vi "OAT Validate Spectrogram Config.vi"(11 "config":T1={"type"=enum."Order-RPM", "range"={"start"=0.0, "end"=0.0, "step"=0.0}} {"range"."step" format="%.2f"; "range"."end" format="%.2f"; "range"."start" format="%.2f"}) -> (3 "config":T1={"type"=enum."Order-RPM", "range"={"start"=0.0, "end"=0.0, "step"=0.0}} {"range"."step" format="%.2f"; "range"."end" format="%.2f"; "range"."start" format="%.2f"})   [LabVIEW 2017, in "SoundVib_Resampling.lvlib"]
uses:
  <vilib>/addons/Sound and Vibration/Order Analysis/Resample Order Tracking/SoundVib_Resampling.lvlib
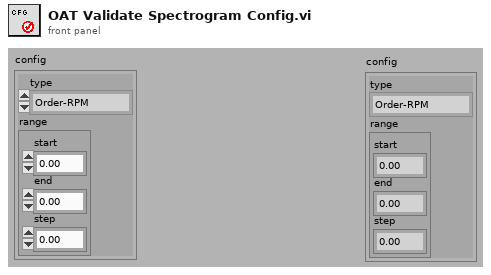
[diagram p1: front panel]
types:
  T1 = cluster{"type":enum16{"Frequency-Time", "Frequency-RPM", "Order-RPM"}, "range":cluster{"start":dbl, "end":dbl, "step":dbl}}
  T2 = enum16{"Frequency-Time", "Frequency-RPM", "Order-RPM"}
  T3 = enum16{"Frequency-Time", "Frequency-RPM", "Order-RPM", "RPM-Order"}
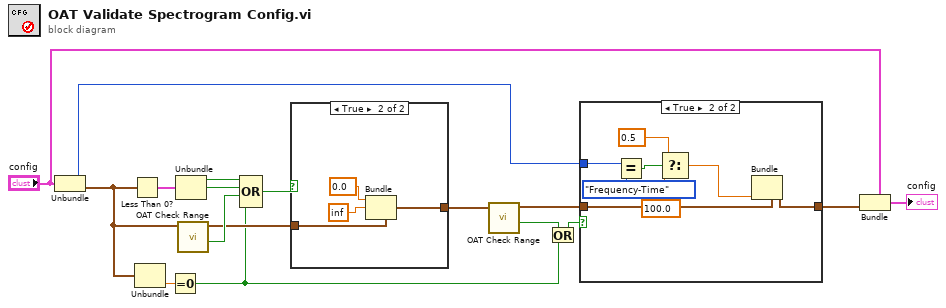
[diagram p0: block diagram]
diagram:
  n1 = Unbundle("config") -> ("type"=w10:T2, "range"=w2:cluster{"start":dbl, "end":dbl, "step":dbl})
  n2 = Less Than 0?(x=w2) -> (x < 0?=w17:cluster{"start":bool, "end":bool, "step":bool})
  n3 = Unbundle(w2) -> ("step"=w6:dbl)  [unwired: 2 out]
  n4 = Equal To 0?(x=w6) -> (x = 0?=w1:bool)
  n5 = Unbundle(w17) -> ("start"=w16:bool, "end"=w15:bool)  [unwired: 1 out]
  n6 = call <vilib>:"OAT Check Range.vi"("range in"=w2) -> ("empty?"=w14:bool, "range out"=w12:cluster{"start":dbl, "end":dbl, "step":dbl})  [unwired: 8 in, 1 out]
  n7 = Compound Arithmetic op=OR(w16, w15, w14, w1) -> (w13:bool)
  n8 = case shown="True" w13 {
    tunnel: w12 -> [w18 w22]
    tunnel: [w18 w19] -> w3
    frame False {
    }
    frame True {
      n9 = Bundle(cluster=w22, "start"=0.0, "end"=inf) -> (w19:cluster{"start":dbl, "end":dbl, "step":dbl})  [unwired: 1 in]
    }
  }
  n10 = call <vilib>:"OAT Check Range.vi"("range in"=w3) -> ("empty?"=w5:bool, "range out"=w11:cluster{"start":dbl, "end":dbl, "step":dbl})  [unwired: 8 in, 1 out]
  n11 = Or(x=w5, y=w1) -> (x .or. y?=w4:bool)
  n12 = case shown="True" w4 {
    tunnel: w11 -> [w23 w26]
    tunnel: [w23 w25] -> w9
    tunnel: w10 -> [_ w30]
    frame False {
    }
    frame True {
      n13 = Equal?(x=w30, y=T3."Frequency-Time") -> (x = y?=w31:bool)
      n14 = Select(t=0.5, s=w31, f=100.0) -> (s? t:f=w24:dbl)
      n15 = Bundle(cluster=w26, "step"=w24) -> (w25:cluster{"start":dbl, "end":dbl, "step":dbl})  [unwired: 2 in]
    }
  }
  n16 = Bundle(cluster="config", "range"=w9) -> (→"config":T1)  [unwired: 1 in]
